vi "Pre-FinalTestBcScan.vi"(11 "error in (no error)":errorcluster, 12 "WAM BarCode":string, 14 "Enable(t)":bool=TRUE) -> (1 "Tested?(t)":bool, 2 "STOP?(t)":bool, 3 "Output String":string="STOP - NO PROGRAMMING DATA\r\nLAST SEEN: N/A\r\nThis module has not been tested before.\r\n", 4 "error?(t)":bool, 15 "error out":errorcluster)   [LabVIEW 2018]
uses:
  Initialize References/Sequence Globals.vi
panel:
  out "py Path":path
  out "Status":string
  out "Message":string
  out "P/F":string="STOP - NO PROGRAMMING DATA"
  out "Array":string[](array[string])
  out "standard error":string
  # "RA24080721"
  # "RGE2100079, 00003609B94D, 2150, B.05, Wideband Antenna Module, 5083561, RaGE Systems, www.ragesystems.com"
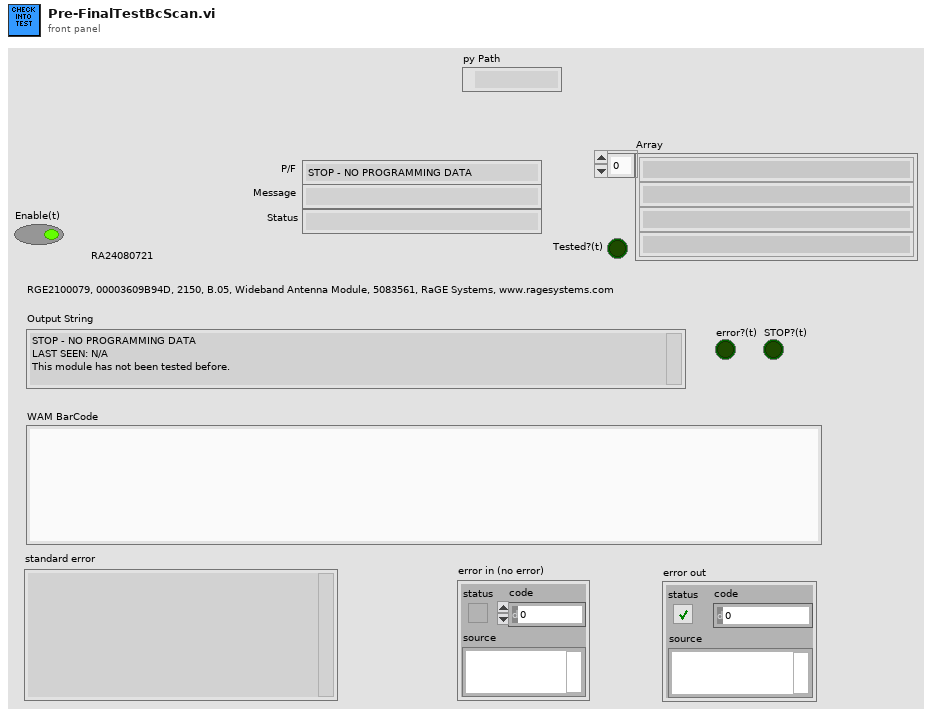
[diagram p1: front panel]
types:
  T1 = enum16{"Left Button", "Center Button", "Right Button", "Window Close"}
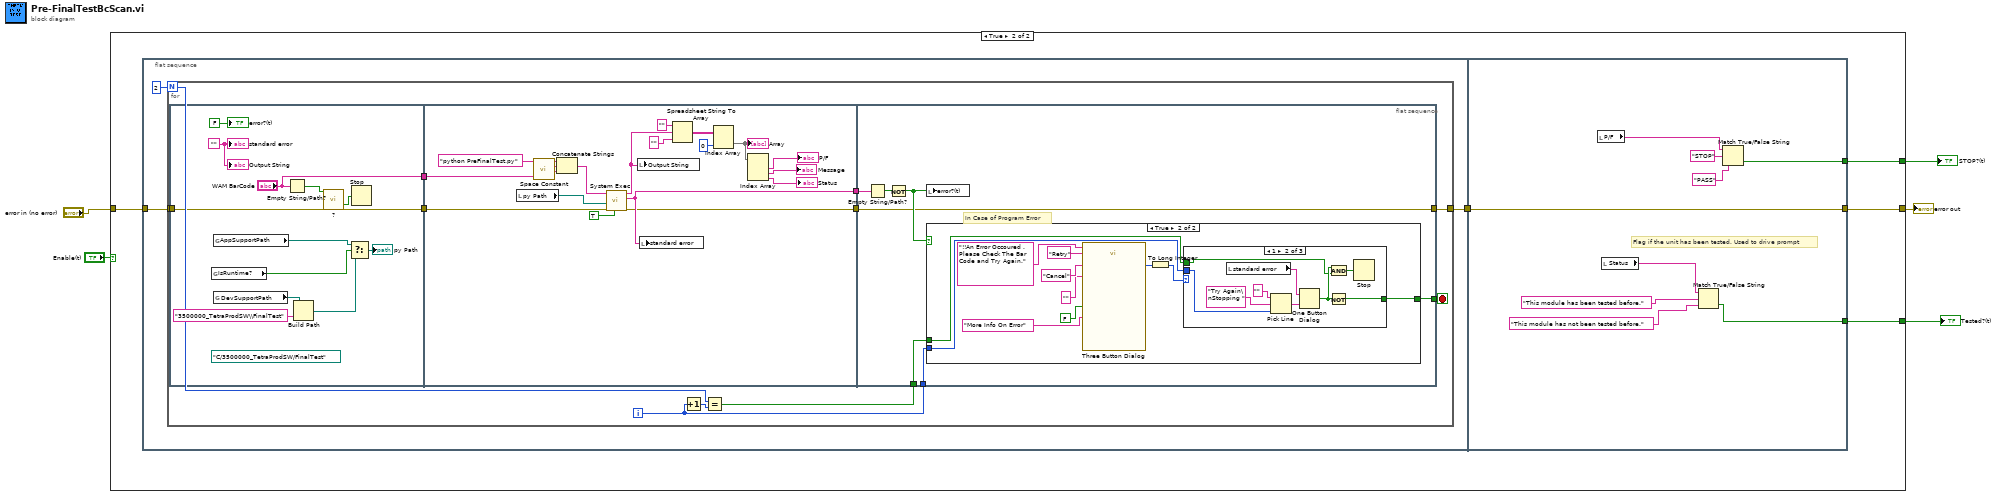
[diagram p0: block diagram]
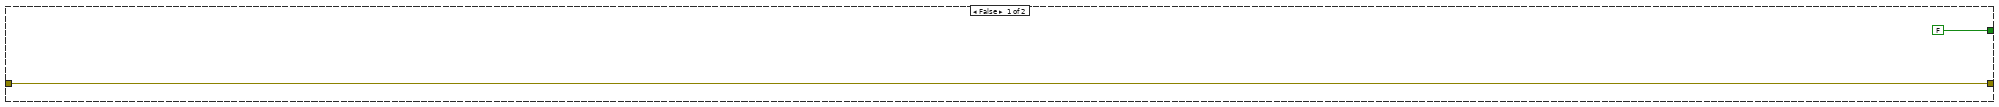
[diagram p2: hidden frame]
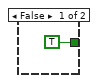
[diagram p3: hidden frame]
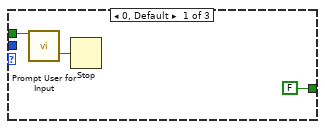
[diagram p4: hidden frame]
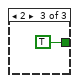
[diagram p5: hidden frame]
diagram:
  n1 = case shown="True" "Enable(t)" {
    tunnel: [w7 w11] -> w5
    tunnel: "error in (no error)" -> [w7 w10]
    tunnel: [FALSE ("selection") w9] -> w2
    tunnel: [_ w8] -> w1
    frame False {
    }
    frame True {
      n2 = flat-sequence {
        tunnel: [w14] -> w12
        tunnel: w10 -> [w13]
        tunnel: [w98] -> w11
        tunnel: w12 -> [w98]
        tunnel: [w94] -> w9
        tunnel: [w90] -> w8
        frame #0 {
          n3 = for {
            N: 2 -> [w23]
            tunnel: [w17] -> w14
            tunnel: w13 -> [w16]
            i -> [w20]
            stop <- w24 stop-if-true
            n4 = flat-sequence {
              tunnel: ["WAM BarCode"] -> w26
              tunnel: [w34] -> w19
              tunnel: w16 -> [w33]
              tunnel: w26 -> [w54]
              tunnel: [w53] -> w25
              tunnel: w19 -> [w51]
              tunnel: [w50] -> w18
              tunnel: w25 -> [w63]
              tunnel: [w62] -> w24
              tunnel: w21 -> [w61]
              tunnel: w20 -> [w60]
              tunnel: [w58] -> w17
              tunnel: w18 -> [w58]
              frame #0 {
                (unwired) path "C:/3500000_TetraProdSW/FinalTest" ("working directory")
                w39 = ""
                n5 = global read "Sequence Globals.vi" "IsRuntime?"() -> (w31:bool)
                n6 = global read "Sequence Globals.vi" "AppSupportPath"() -> (w32:path)
                n7 = global read "Sequence Globals.vi" "DevSupportPath"() -> (w29:path)
                n8 = Empty String/Path?(string/path="WAM BarCode") -> (empty?=w37:bool)
                n9 = Build Path(base path=w29, name or relative path="3500000_TetraProdSW\\FinalTest") -> (appended path=w28:path)
                n10 = call "?"("Enable"=w37, "error in (no error)"=w33) -> ("OK"=w36:bool, "error out"=w34:errorcluster)  [unwired: 16 in]
                n11 = Select(t=w32, s=w31, f=w28) -> (s? t:f=→"py Path":path)
                n12 = Stop(stop? (T)=w36) -> ()
                "Output String" <- w39
                "standard error" <- w39
                "error?(t)" <- FALSE ("error?(t)")
              }
              frame #1 {
                n13 = local read "py Path"() -> (w40:path)
                n14 = call <vilib>:"Space Constant.vi"() -> ("String"=w55:string)
                n15 = Concatenate Strings("python PreFinalTest.py" ("command line"), w55, w54) -> (w56:string)
                n16 = call <vilib>:"System Exec.vi"("run minimized? (F)"=TRUE, "error in (no error)"=w51, "working directory"=w40, "command line"=w56) -> ("error out"=w50:errorcluster, "standard error"=w53:string, "standard output"=w49:string)  [unwired: 4 in, 1 out]
                n17 = local write "Output String"(w49) -> ()
                n18 = local write "standard error"(w53) -> ()
                n19 = Spreadsheet String To Array(format string="", spreadsheet string=w49, array type (2D Dbl)="") -> (array=w46:string[][])  [unwired: 1 in]
                n20 = Index Array(array=w46, index (col)=0 ("disabled index (col)")) -> (element=w44:string[])  [unwired: 1 in]
                "Array" <- w44
                n21 = Index Array(array=w44) -> (element #1=→"P/F":string, element #2=→"Message":string, element #3=→"Status":string)  [unwired: 3 in]
              }
              frame #2 {
                # "In Case of Program Error"
                n22 = Empty String/Path?(string/path=w63) -> (empty?=w64:bool)
                n23 = Not(x=w64) -> (.not. x?=w59:bool)
                n24 = local write "error?(t)"(w59) -> ()
                n25 = case shown="True" w59 {
                  tunnel: [TRUE w68] -> w62
                  tunnel: w61 -> [_ w67]
                  tunnel: w60 -> [_ w66]
                  frame False {
                  }
                  frame True {
                    n26 = call <vilib>:"Three Button Dialog.vi"("Allow user to close window? (TRUE)"=FALSE, "Window Title (\"\")"="" ("Window Title (\"\")"), "Right Button Text (\"Cancel\")"="Cancel" ("Right Button Text (\"Cancel\")"), "Center Button Text (\"No\")"="More Info On Error" ("Center Button Text (\"No\")"), "Left Button Text (\"Yes\")"="Retry" ("Left Button Text (\"Yes\")"), "message"="!!An Error Occoured . Please Check The Bar Code and Try Again." ("Message")) -> ("Which Button?"=w70:T1)  [unwired: 5 in]
                    n27 = To Long Integer(number=w70) -> (32bit integer=w69:i32)
                    n28 = case shown="1" w69 {
                      tunnel: [FALSE w87 TRUE] -> w68
                      tunnel: w67 -> [w78 w85 _]
                      tunnel: w66 -> [_ w80 _]
                      frame 0, Default {
                        n29 = call "Prompt User for Input"("Enable"=w78) -> ("OK"=w77:bool)  [unwired: 17 in, 1 out]
                        n30 = Stop(stop? (T)=w77) -> ()
                      }
                      frame 1 {
                        n31 = local read "standard error"() -> (w88:string)
                        n32 = Pick Line(string ("")="", multi-line string="Try Again\nStopping " ("button name (\"OK\")"), line index=w80) -> (output string=w83:string)
                        n33 = One Button Dialog(message=w88, button name ("OK")=w83) -> (true=w86:bool)
                        n34 = Not(x=w86) -> (.not. x?=w87:bool)
                        n35 = And(x=w86, y=w85) -> (x .and. y?=w84:bool)
                        n36 = Stop(stop? (T)=w84) -> ()
                      }
                      frame 2 {
                      }
                    }
                  }
                }
              }
            }
            n37 = Increment(x=w20) -> (x+1=w22:i32)
            n38 = Equal?(x=w23, y=w22) -> (x = y?=w21:bool)
          }
        }
        frame #1 {
          # "Flag if the unit has been tested. Used to drive prompt"
          n39 = local read "P/F"() -> (w97:string)
          n40 = local read "Status"() -> (w93:string)
          n41 = Match True/False String(2:"This module has not been tested before." ("regular expression"), 3:"This module has been tested before." ("regular expression"), 4:w93) -> (0:w90:bool)  [unwired: 1 out]
          n42 = Match True/False String(2:"PASS" ("true string"), 3:"STOP" ("false string"), 4:w97) -> (0:w94:bool)  [unwired: 1 out]
        }
      }
    }
  }
  "error out" <- w5
  "STOP?(t)" <- w2
  "Tested?(t)" <- w1
